vi "New Lua State.vi"(6 "open libs? (T)":bool=TRUE, 8 "error in (no error)":errorcluster) -> (0 "error out":errorcluster, 3 "Lua out":refnum<data-value>)   [LabVIEW 2020, in "Lua for LabVIEW.lvlib" / "Lua.lvclass"]
doc: "Creates a new Lua state. \n\nDefaults to open all standard Lua libraries."
uses:
  Lua.lvclass
  private/lua_monitor_event.ctl
  Lua.lvclass/Lua.ctl
  private/lua_monitor.vi
  lib/lua.dll/lua.dll.lvlib
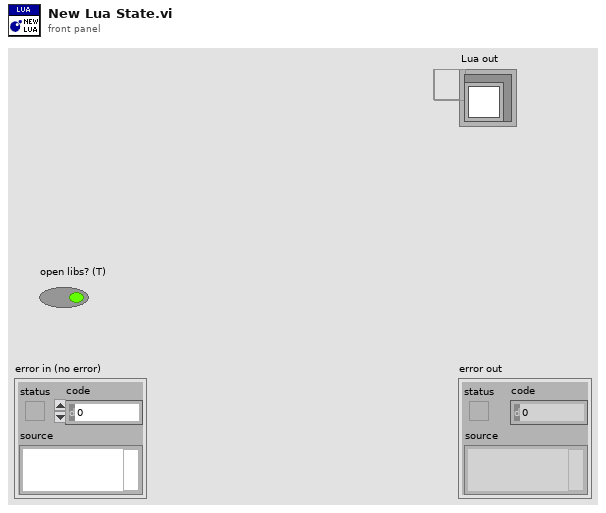
[diagram p1: front panel]
types:
  T1 = typedef "Lua for LabVIEW.lvlib/Lua.lvclass/lua_monitor_event.ctl" = enum16{"<null>", "terminate"}
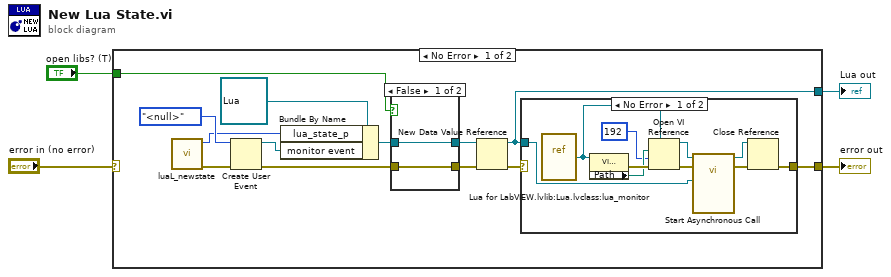
[diagram p0: block diagram]
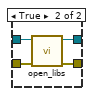
[diagram p2: hidden frame]
diagram:
  n1 = case shown="No Error" "error in (no error)" {
    selector: "error in (no error)" -> [_ w35]
    tunnel: [w11 w35] -> w3
    tunnel: [w10 _] -> w2
    tunnel: "open libs? (T)" -> [w5 _]
    frame No Error {
      n2 = call "luaL_newstate.vi"() -> ("error out"=w14:errorcluster, "lua_state_p"=w15:u64)  [unwired: 10 in]
      n3 = Create User Event(user event datatype=lua_monitor_event."<null>" ("event"), error in=w14) -> (user event=w13:refnum<user-event>, error out=w6:errorcluster)
      n4 = Bundle By Name(cluster=refnum<class "Lua.lvclass"> refnum ("Lua in"), "lua_state_p"=w15, "monitor event"=w13) -> (w9:refnum<class "Lua.lvclass">)
      n5 = case shown="False" w5 {
        tunnel: w9 -> [w19 w23]
        tunnel: [w19 w22] -> w8
        tunnel: [w18 w21] -> w7
        tunnel: w6 -> [w18 w20]
        frame False {
        }
        frame True {
          n6 = call-dynamic "open_libs.vi"("error in (no error)"=w20, "Lua in"=w23) -> ("error out"=w21:errorcluster, "Lua out"=w22:refnum<class "Lua.lvclass">)  [unwired: 8 in]
        }
      }
      n7 = New Data Value Reference(data value=w8, error in=w7) -> (data value reference=w10:refnum<data-value>, error out=w12:errorcluster)
      n8 = case shown="No Error" w12 {
        selector: w12 -> [_ w34]
        tunnel: [w24 w34] -> w11
        tunnel: w10 -> [w27 _]
        frame No Error {
          n9 = vi-ref "Lua for LabVIEW.lvlib:Lua.lvclass:lua_monitor.vi"() -> (w32:refnum<vi>)
          n10 = property class="VI (strict)"(reference=w32) -> (error out=w33:errorcluster, "Path"=w31:path)  [unwired: 1 in, 1 out]
          n11 = Open VI Reference(type specifier VI Refnum (for type only)=w32, vi path=w31, options=192, error in (no error)=w33) -> (vi reference=w29:refnum<vi>, error out=w28:errorcluster)  [unwired: 2 in]
          n12 = call-by-ref "Start Asynchronous Call"(reference=w29, error in=w28, "Lua for LabVIEW.lvlib:Lua.lvclass"=w27) -> (reference out=w26:refnum<vi>, error out=w25:errorcluster)  [unwired: 11 in]
          n13 = Close Reference(reference=w26, error in (no error)=w25) -> (error out=w24:errorcluster)
        }
        frame Error {
        }
      }
    }
    frame Error {
    }
  }
  "error out" <- w3
  "Lua out" <- w2
